vi "Set PrePurgePrintCount_StatusChangedEvent.vi"(8 "error in (no error)":errorcluster, 10 "Status.PrePurgePrintNo":i32, 11 "TopLevel in":refnum<class "TopLevel.lvclass">) -> (0 "error out":errorcluster, 3 "TopLevel out":refnum<class "TopLevel.lvclass">)   [LabVIEW 2022 SP3, in "TopLevel.lvclass"]
uses:
  TopLevel.lvclass
  TopLevel.lvclass/TopLevel.ctl
  Motor Controller/Motor Controller.lvclass
  IO/IO.lvclass
  GIS Printer/GIS Printer.lvclass
  Database/Database.lvclass
  DLP2/DLP2.lvclass
  DAQWFE/LV_Source/Subsystems/DAQ/DAQ.lvclass
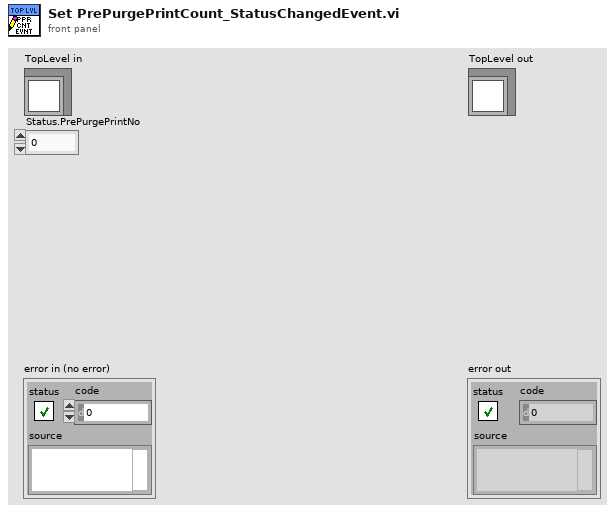
[diagram p1: front panel]
types:
  T1 = typedef "TopLevel.lvclass/Private Data.ctl" = cluster{"UserEvents":T2, "All Dependencies":cluster{"Class References":refnum<class>[], "Class Names":string[]}, "Motor Controller Obj":refnum<class "Motor Controller.lvclass">, "IO Obj":refnum<class "IO.lvclass">, "Laser Obj":refnum<class "GIS Printer.lvclass">, "Digilens IPLC Config":T3, "Status":T14, "Database Obj":refnum<class "Database.lvclass">, "DLP2 Obj":refnum<class "DLP2.lvclass">, "MasterConfigurationDLPC2":T15, "DAQ":refnum<class "DAQ.lvclass">, "ConfigDIct":T23, "DLP":T24, "PersistentData":T31, "UserLevel":T32, "ProcessMode":T33, "Str Refnum":refnum<vi>}
  T2 = typedef "TopLevel.lvclass/UserEvents.ctl" = cluster{"API Incoming Event":refnum<user-event>, "API Executed Event":refnum<user-event>, "API Return Event":refnum<user-event>, "Exit Event":refnum<user-event>, "StatusChanged":refnum<user-event>, "DLP GUI Config Changed":refnum<user-event>, "AppEvent":refnum<user-event>, "Login Event":refnum<user-event>, "HeadPrimeStatusEvent":refnum<user-event>}
  T3 = typedef "TopLevel.lvclass/Digilens Config Cluster.ctl" = cluster{"Motion Controller":T4, "IO Config":T5, "PrinterConfiguration":T8, "DAQ Settings":T9}
  T4 = typedef "Motor Controller.lvclass/Motor Controller Config Data.ctl" = cluster{"Motor IP Addresss":string, "Current Position":i32, "Pulse_Per_mm":i32, "PrePrint":dbl[], "Load Position_mm":i32, "Laminate Position_mm":i32}
  T5 = typedef "IO.lvclass/IO Config Data.ctl" = cluster{"DAQDevices":T6[], "DI Channels":T7[], "DO Channels":T7[], "Material Names":string[], "AI Channels":T7[], "AO Channels":T7[]}
  T6 = typedef "IO.lvclass/DCON_DeviceConfig--Cluster.ctl" = cluster{"COM":string, "DeviceName":string, "BaudRate":u32, "Number of Channels":i32, "DeviceAddress":i32, "Enable":bool}
  T7 = typedef "IO.lvclass/Channel Data.ctl" = cluster{"Channel Name":string, "Device Name":string, "Channel No":string}
  T8 = typedef "GIS Printer.lvclass/PrinterConfiguration--Cluster.ctl" = cluster{"IPAddress":string, "Move Stage on RTP Command?":bool, "Stage Move Position":string, "PH1-Prime Path":path, "PH2-Prime Path":path, "PH3-Prime Path":path, "PH4-Prime Path":path, "PH5-Prime Path":path, "PH6-Prime Path":path, "PrintScriptsFolder":path, "PurgeScriptsFolder":path, "StageScriptsFolder":path, "PH1-HeatOn Path":path, "PH2-HeatOn Path":path, "PH3-HeatOn Path":path, "PH4-HeatOn Path":path, "PH5-HeatOn Path":path, "PH6-HeatOn Path":path, "PH1-HeatOff Path":path, "PH2-HeatOff Path":path, "PH3-HeatOff Path":path, "PH4-HeatOff Path":path, "PH5-HeatOff Path":path, "PH6-HeatOff Path":path}
  T9 = typedef "DAQ.lvclass/TD DAQ Settings--cluster.ctl" = cluster{"Simulate DAQ":bool, "DI Settings":T10[], "AI Settings":T11[], "Relay IONames":string[], "AO IONames":string[], "AO NChan SingleTask":bool}
  T10 = typedef "DAQ.lvclass/TD DI Instrument Settings--cluster.ctl" = cluster{"Disable":bool, "DI TaskName":string, "DI RefreshIntv":i32}
  T11 = typedef "DAQ.lvclass/TD AI Instrument Settings--cluster.ctl" = cluster{"Disable":bool, "AI TaskName":string, "AI InstSettings":T12, "SimAI Ranges":T13}
  T12 = typedef "DAQ.lvclass/TD AI InstSettings--cluster.ctl" = cluster{"DaqRate":dbl, "NumSamples":i32}
  T13 = typedef "DAQ.lvclass/TD SimAI Ranges--cluster.ctl" = cluster{"lo":dbl, "hi":dbl}
  T14 = typedef "Status_TopLevel--Cluster.ctl" = cluster{"Busy":bool, "Time":timestamp, "error":errorcluster, "PrintNo":i32, "PrePurgePrintNo":i32, "CalPrintNo":i32}
  T15 = typedef "TD MasterConfiguration DLPC2--cluster.ctl" = cluster{"Paths":T16, "ColorPaneMapping":T17, "Materials":string[], "ColorPlanes":string[], "SpitVoltages_Half":T19, "SpitVoltages_Full":T19, "SystemMode":string[], "PrimeModeConfig":T20[], "Running Average Duration_s":dbl}
  T16 = typedef "DLPC2_Path--Cluster.ctl" = cluster{"DigiBit WG Design Folder":path, "Compensated GS Image Folder":path, "Nozzle GS Files Head 1":path, "Nozzle GS Files Head 2":path, "Nozzle GS Files Head 3":path, "Nozzle GS Files Head 4":path, "Nozzle GS Files Head 5":path, "Nozzle GS Files Head 6":path}
  T17 = typedef "TD HeadColorPaneMappingAll--cluster.ctl" = cluster{"Head 1":T18, "Head 2":T18, "Head 3":T18, "Head 4":T18, "Head 5":T18, "Head 6":T18}
  T18 = typedef "TD HeadColorPaneMapping--cluster.ctl" = cluster{"Material":string, "ColorPane":string}
  T19 = typedef "SpitVoltages--Cluster.ctl" = cluster{"1":dbl, "2":dbl, "3":dbl, "4":dbl, "5":dbl, "6":dbl}
  T20 = typedef "TopLevel.lvclass/PrimingMode APIData.ctl" = cluster{"Interval (s)":dbl, "PurgeDuration (s)":dbl, "Repeats":u8, "PrimingMode":T21, "Head":T22, "Frequency (Hz)":i32, "PrintWeight":dbl}
  T21 = typedef "PurgeMode--Enum.ctl" = enum16{"Pre-Purge", "Purge", "Spit", "Shake"}
  T22 = typedef "PrinterHeads--Enum.ctl" = enum16{"-1", "1", "2", "3", "4", "5", "6"}
  T23 = typedef "TD Dynamic CVT DVR--ref.ctl" = refnum<data-value>
  T24 = typedef "DLPConfig_Initialization.ctl" = cluster{"PrinterInitialization":cluster{"Printer":cluster{"#attributes":cluster{"Name":string}}, "VacPumpSet":cluster{"#attributes":cluster{"VacPumpEnable":bool, "VacPumpSpeed":dbl}}, "HIBEnable":cluster{"#attributes":cluster{"HIB1Enable":bool, "HIB2Enable":bool, "HIB3Enable":bool, "HIB4Enable":bool, "HIB5Enable":bool, "HIB6Enable":bool}}, "PrinterCompensation":T25}, "HeadSet":cluster{"HeadProperties":T26[]}, "InkSet":cluster{"Ink":T28[]}, "Troubleshooting":cluster{"PMBLogging":cluster{"#attributes":cluster{"PMBMonitorDuringPrint":bool, "PMBMonitorDuringIdle":bool, "LogSwatheInputData":bool, "LogSwatheOutputData":bool, "LogPrintheadColourPlanes":bool, "LogPMBCommunication":bool, "LogSimulatedOutput":bool, "LogAllPMBCommunicationData":bool, "LogPMBSpace":bool, "ExtendedPMBSpaceLogging":bool, "LogPMBWriteSpeed":bool, "LogUsbRetries":bool}}, "HIBLogging":cluster{"#attributes":cluster{"HIBMonitoringDuringPrint":bool, "HIBMonitoringLog":bool}}}}
  T25 = typedef "DLP2_PrinterCompensationProperties.ctl" = cluster{"#attributes":cluster{"AppName":string, "PrintWeightMultiplier":dbl, "Rotation":bool, "Driver":string, "Server":string, "Database":string, "User":string, "Password":string}}
  T26 = typedef "DLP2_PrinterHeadProperties.ctl" = cluster{"#attributes":T27}
  T27 = typedef "DLPConfig)Init_HeadPropertyAttr--Cluster.ctl" = cluster{"HeadNumber":u8, "Material":string, "HeadLocalX":dbl, "HeadLocalY":dbl, "HeadRotationAngle":dbl, "VH2L_Hi":dbl, "VH2R_Hi":dbl, "VH1LA_Hi":dbl, "VH1LB_Hi":dbl, "VH1RA_Hi":dbl, "VH1RB_Hi":dbl, "VH2L_Lo":dbl, "VH2R_Lo":dbl, "VH1LA_Lo":dbl, "VH1LB_Lo":dbl, "VH1RA_Lo":dbl, "VH1RB_Lo":dbl}
  T28 = typedef "DLP2_PrinterMaterialProperties.ctl" = cluster{"#attributes":cluster{"InkType":string, "ColorPlane":string, "PrePrintPurge":bool, "PurgeTime":dbl, "PurgeCount":i32, "Density":dbl, "NumberofDrops":i32, "PrintWeight":dbl, "PrintheadPrime":bool}, "Idle":T29, "Process":T30}
  T29 = typedef "InkIdleNodeConfigXML--Cluster.ctl" = cluster{"ShortIdle":cluster{"#attributes":cluster{"Heat":dbl, "Meniscus":dbl, "Recirculation":bool}}, "LongIdle":cluster{"#attributes":cluster{"Heat":dbl, "Meniscus":dbl, "Recirculation":bool}}}
  T30 = typedef "InkProcessNodeConfigXML--Cluster.ctl" = cluster{"C30_Process":cluster{"#attributes":cluster{"Heat":dbl, "Meniscus":dbl, "Recirculation":bool, "ColorPlane":string}}, "S30_Process":cluster{"#attributes":cluster{"Heat":dbl, "Meniscus":dbl, "Recirculation":bool, "ColorPlane":string}}}
  T31 = typedef "PersistentData--Cluster.ctl" = cluster{"ToolIdle":bool, "Meniscus Vac Pump Speed":dbl, "InkChEnable":cluster{"Enable Ink Ch-1":bool, "Enable Ink Ch-2":bool, "Enable Ink Ch-3":bool, "Enable Ink Ch-4":bool, "Enable Ink Ch-5":bool, "Enable Ink Ch-6":bool}, "HeatEnable":cluster{"Heater-1 Off":bool, "Heater-2 Off":bool, "Heater-3 Off":bool, "Heater-4 Off":bool, "Heater-5 Off":bool, "Heater-6 Off":bool}, "MiniscusPressure":cluster{"Meniscus Pressure Set - R1":dbl, "Meniscus Pressure Set - R2":dbl, "Meniscus Pressure Set - R3":dbl, "Meniscus Pressure Set - R4":dbl, "Meniscus Pressure Set - R5":dbl, "Meniscus Pressure Set - R6":dbl}, "RecircPumpFlow":cluster{"Recirc Pump Flow Set - R1":dbl, "Recirc Pump Flow Set - R2":dbl, "Recirc Pump Flow Set - R3":dbl, "Recirc Pump Flow Set - R4":dbl, "Recirc Pump Flow Set - R5":dbl, "Recirc Pump Flow Set - R6":dbl}}
  T32 = typedef "UserLevel--Enum.ctl" = enum16{"None", "Operator", "Engineer"}
  T33 = typedef "processMode--enum.ctl" = enum16{"Short Idle", "Long Idle ", "C30_Process", "S30_Process"}
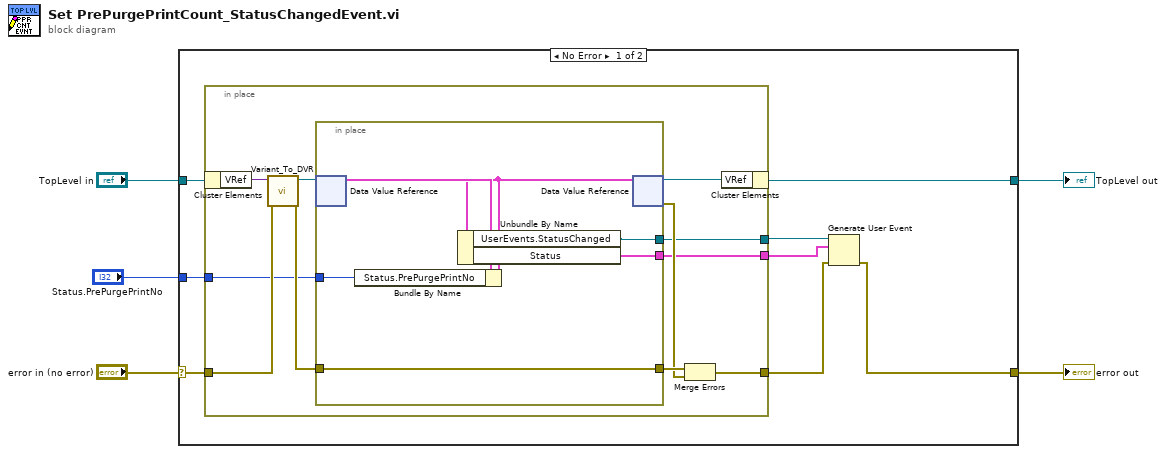
[diagram p0: block diagram]
diagram:
  n1 = case shown="No Error" "error in (no error)" {
    selector: "error in (no error)" -> [w11 w32]
    tunnel: [w6 w32] -> w3
    tunnel: [w13 w31] -> w2
    tunnel: "TopLevel in" -> [w12 w31]
    tunnel: "Status.PrePurgePrintNo" -> [w10 _]
    frame No Error {
      n2 = in-place {
        in-place-border: w11 -> [w22]
        in-place-border: [w18] -> w7
        in-place-border: w10 -> [w16]
        in-place-border: [w15] -> w9
        in-place-border: [w14] -> w8
        n3 = in-place-cluster #1(w12) -> ("VRef"=w24:variant)
        n4 = call "Variant_To_DVR.vi"("error in (no error)"=w22, "Variant"=w24) -> ("error out"=w21:errorcluster, "DVR"=w23:refnum<data-value>)  [unwired: 8 in]
        n5 = in-place {
          in-place-border: w21 -> [w30]
          in-place-border: [w30] -> w20
          in-place-border: w16 -> [w28]
          in-place-border: [w26] -> w15
          in-place-border: [w25] -> w14
          n6 = in-place-dvr #2(w23) -> (w29:T1)  [unwired: 1 out]
          n7 = Bundle By Name(cluster=w29, "Status.PrePurgePrintNo"=w28) -> (w27:T1)
          n8 = Unbundle By Name(w27) -> ("UserEvents.StatusChanged"=w26:refnum<user-event>, "Status"=w25:T14)
          n9 = in-place-dvr #2(w27) -> (w17:refnum<data-value>, w19:errorcluster)
        }
        n10 = Merge Errors(w20, w19) -> (w18:errorcluster)
        n11 = in-place-cluster #1("VRef"=w17) -> (w13:refnum<class "TopLevel.lvclass">)
      }
      n12 = Generate User Event(user event=w9, event data cluster=w8, error in=w7) -> (error out=w6:errorcluster)  [unwired: 1 in, 1 out]
    }
    frame Error {
    }
  }
  "error out" <- w3
  "TopLevel out" <- w2
